vi "List Measurement Parameters.vi"(8 "Error In (no error)":errorcluster, 10 "Channel (1)":i32=1, 11 "VISA Resource Name":refnum<visa-resource-name>) -> (0 "Error Out":errorcluster, 2 "Measurement Parameter Array":string[][](array[string]), 3 "VISA Resource Name Out":refnum<visa-resource-name>)   [LabVIEW 2014, in "Agilent PNA Series.lvlib"]
doc: "This VI returns a string array of valid analyzer measurement parameters for the selected channel."
uses:
  Agilent PNA Series.lvlib
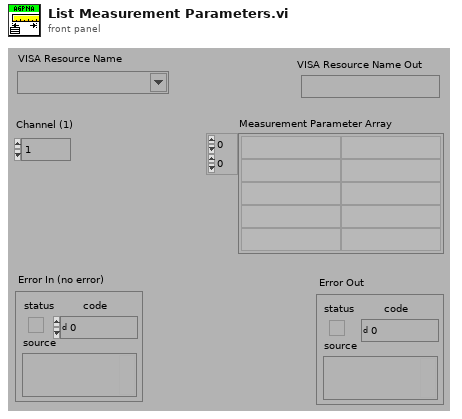
[diagram p1: front panel]
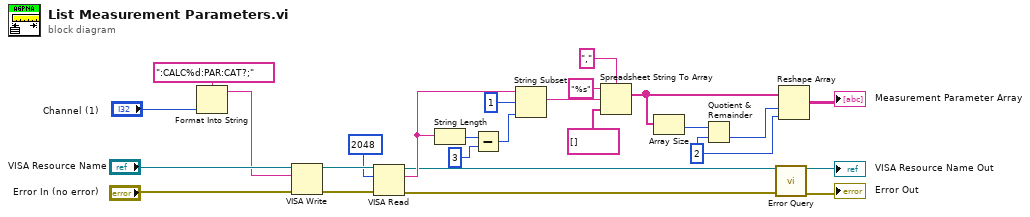
[diagram p0: block diagram]
diagram:
  w7 = 2 ("dimension size")
  n1 = Format Into String(format string=":CALC%d:PAR:CAT?;", "Channel (1)") -> (resulting string=w5:string)  [unwired: 2 in, 1 out]
  n2 = VISA Write(VISA resource name="VISA Resource Name", write buffer=w5, error in (no error)="Error In (no error)") -> (VISA resource name out=w23:refnum<visa-resource-name>, error out=w22:errorcluster)  [unwired: 1 out]
  n3 = VISA Read(VISA resource name=w23, byte count=u32 2048 ("byte count (0)"), error in (no error)=w22) -> (VISA resource name out=w4:refnum<visa-resource-name>, read buffer=w11:string, error out=w3:errorcluster)  [unwired: 1 out]
  n4 = String Length(string=w11) -> (length=w14:i32)
  n5 = Subtract(x=w14, y=3) -> (x-y=w12:i32)
  n6 = String Subset(string=w11, offset (0)=1, length (rest)=w12) -> (substring=w16:string)
  n7 = Spreadsheet String To Array(delimiter (Tab)=",", format string="%s", spreadsheet string=w16, array type (2D Dbl)=string[] []) -> (array=w9:string[])
  n8 = Array Size(array=w9) -> (size(s)=w8:i32)
  n9 = Quotient & Remainder(x=w8, y=w7) -> (floor(x/y)=w6:i32)  [unwired: 1 out]
  n10 = call "Error Query.vi"("VISA Resource Name"=w4, "error in (no error)"=w3) -> ("VISA Resource Name Out"=→"VISA Resource Name Out":refnum<visa-resource-name>, "error out"=→"Error Out":errorcluster)  [unwired: 10 in, 2 out]
  n11 = Reshape Array(w9, w6, w7) -> (→"Measurement Parameter Array":string[][])
